vi "Trigger Pruefen.vi"(9 "Triggerereignis":T1 {"kl./gr." items=["kleiner", "größer"]; "Trigger verwenden" items=["Deaktiviert", "Aktiviert"]}) -> (1 "Trigger":bool)   [LabVIEW 2020, in "LogKonfig.lvlib"]
uses:
  LogKonfig.lvlib
  Element Triggerereignisse.ctl
  Auswahlfeld aktiviert-deaktiviert.ctl
  Messdaten/Aktionen FGV Messdaten.ctl
  Messdaten/Messdaten.lvlib
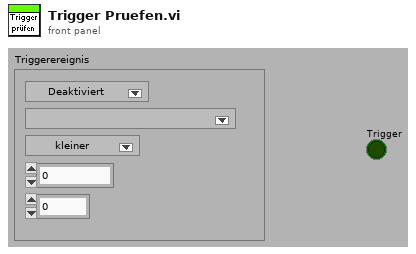
[diagram p1: front panel]
types:
  T1 = typedef "LogKonfig.lvlib/Element Triggerereignisse.ctl" = cluster{"Trigger verwenden":T2, "Messwert":u16, "kl./gr.":u16, "Wert":sgl, "Puffergröße":sgl}
  T2 = typedef "LogKonfig.lvlib/Auswahlfeld aktiviert-deaktiviert.ctl" = u16
  T3 = typedef "Messdaten.lvlib/Aktionen FGV Messdaten.ctl" = enum16{"lesen", "schreiben", "löschen", "Mittelwerte", "Komponente"}
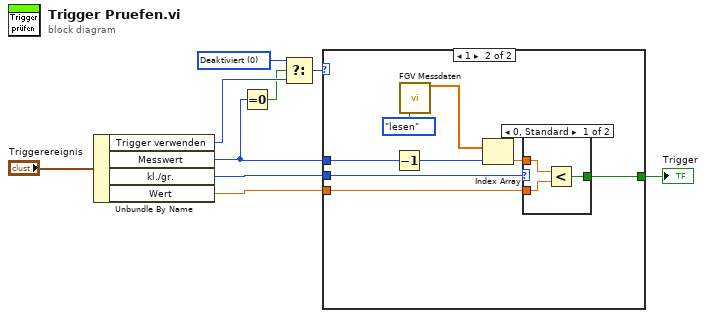
[diagram p0: block diagram]
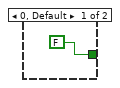
[diagram p2: hidden frame]
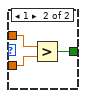
[diagram p3: hidden frame]
diagram:
  w1 = T2 0 items=["Deaktiviert", "Aktiviert"] ("t")
  n1 = Unbundle By Name("Triggerereignis") -> ("Trigger verwenden"=w5:T2, "Messwert"=w2:u16, "kl./gr."=w8:u16, "Wert"=w7:sgl)
  n2 = Equal To 0?(x=w2) -> (x = 0?=w3:bool)
  n3 = Select(t=w1, s=w3, f=w5) -> (s? t:f=w4:T2)
  n4 = case shown="1" w4 {
    tunnel: w2 -> [_ w12]
    tunnel: w8 -> [_ w18]
    tunnel: w7 -> [_ w16]
    tunnel: [FALSE w15] -> w6
    frame 0, Default {
    }
    frame 1 {
      n5 = Decrement(x=w12) -> (x-1=w11:u16)
      n6 = call "FGV Messdaten.vi"("Aktionen"=Aktionen_FGV_Messdaten."lesen") -> ("Aktuelle Messwerte"=w13:sgl[])  [unwired: 6 in, 8 out]
      n7 = Index Array(array=w13, index=w11) -> (element=w17:sgl)
      n8 = case shown="0, Standard" w18 {
        tunnel: w17 -> [w21 w24]
        tunnel: w16 -> [w20 w23]
        tunnel: [w19 w22] -> w15
        frame 0, Default {
          n9 = Less?(x=w21, y=w20) -> (x < y?=w19:bool)
        }
        frame 1 {
          n10 = Greater?(x=w24, y=w23) -> (0:w22:bool)
        }
      }
    }
  }
  "Trigger" <- w6
